vi "Notify.vi"(8 "error in (no error)":errorcluster, 10 "ErrorOrSuccess":refnum<class "ErrorOrSuccess.lvclass">, 11 "IRegister in":refnum<class "IRegister.lvclass">) -> (0 "error out":errorcluster, 3 "IRegister out":refnum<class "IRegister.lvclass">)   [LabVIEW 2020, in "wamplv.lvlib" / "IRegister.lvclass"]
uses:
  IRegister.lvclass
  Message loop classes/ErrorOrSuccess/ErrorOrSuccess.lvclass
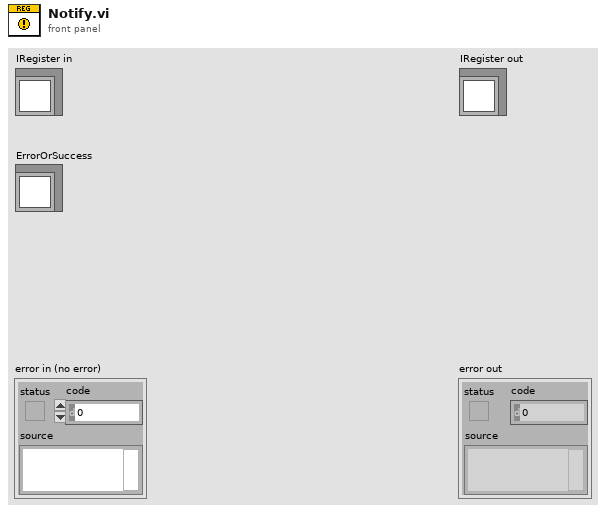
[diagram p1: front panel]
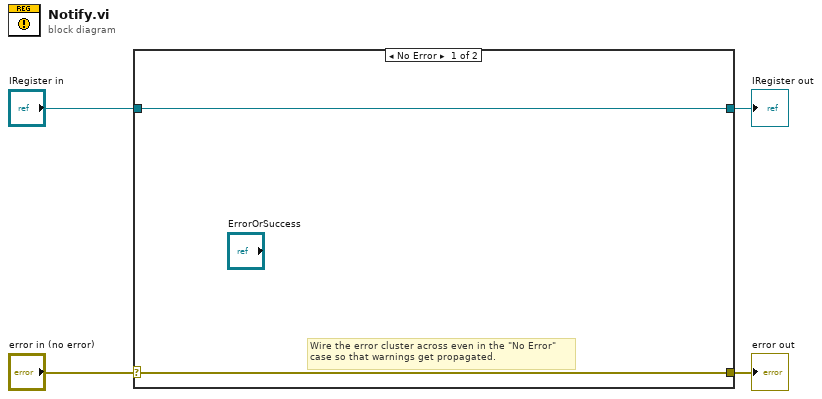
[diagram p0: block diagram]
diagram:
  n1 = case shown="No Error" "error in (no error)" {
    selector: "error in (no error)" -> [w5 w8]
    tunnel: [w5 w8] -> w3
    tunnel: [w6 w7] -> w1
    tunnel: "IRegister in" -> [w6 w7]
    frame No Error {
      # "Wire the error cluster across even in the \"No Error\"\ncase so that warnings get propagated."
    }
    frame Error {
    }
  }
  "error out" <- w3
  "IRegister out" <- w1
